vi "Add Node to Children.vi"(9 "Parent Path":string, 10 "Node Path":string, 11 "Tree Map In":T1) -> (1 "Path Invalid":bool, 3 "Tree Map Out":T1)   [LabVIEW 2019, in "Tree Map.lvlib"]
doc: "<b>Author:</b> Piotr Kruczkowski <PrimaryKey>\n<b>License:</b> NewBSD\n\nCopyright (c) 2019, National Instruments\nAll rights reserved.\n\nRedistribution and use in source and binary forms, with or without\nmodification, are permitted provided that the following conditions are met:\n1. Redistributions of source code must retain the above copyright\n notice, this list of conditions and the following disclaimer.\n2. Redistributions in binary form must reproduce the above copyright\n notice, this list of conditions and the following disclaimer in the\n documentation and/or other materials provided with the distribution.\n3. Neither the name of National Instruments nor the\n names of its contributors may be used to endorse or promote products\n derived from this software without specific prior written permission.\n\nTHIS SOFTWARE IS PROVIDED BY National Instruments ''AS IS'' AND ANY\nEXPRESS OR IMPLIED WARRANTIES, INCLUDING, BUT NOT LIMITED TO, THE IMPLIED\nWARRANTIES OF MERCHANTABILITY AND FITNESS FOR A PARTICULAR PURPOSE ARE\nDISCLAIMED. IN NO EVENT SHALL National Instruments BE LIABLE FOR ANY\nDIRECT, INDIRECT, INCIDENTAL, SPECIAL, EXEMPLARY, OR CONSEQUENTIAL DAMAGES\n(INCLUDING, BUT NOT LIMITED TO, PROCUREMENT OF SUBSTITUTE GOODS OR SERVICES;\nLOSS OF USE, DATA, OR PROFITS; OR BUSINESS INTERRUPTION) HOWEVER CAUSED AND\nON ANY THEORY OF LIABILITY, WHETHER IN CONTRACT, STRICT LIABILITY, OR TORT\n(INCLUDING NEGLIGENCE OR OTHERWISE) ARISING IN ANY WAY OUT OF THE USE OF THIS\nSOFTWARE, EVEN IF ADVISED OF THE POSSIBILITY OF SUCH DAMAGE."
uses:
  Tree Map.lvlib
  Tree Map Data.ctl
  <vilib>/Utility/miscctls.llb/LVMapReplaceAction.ctl
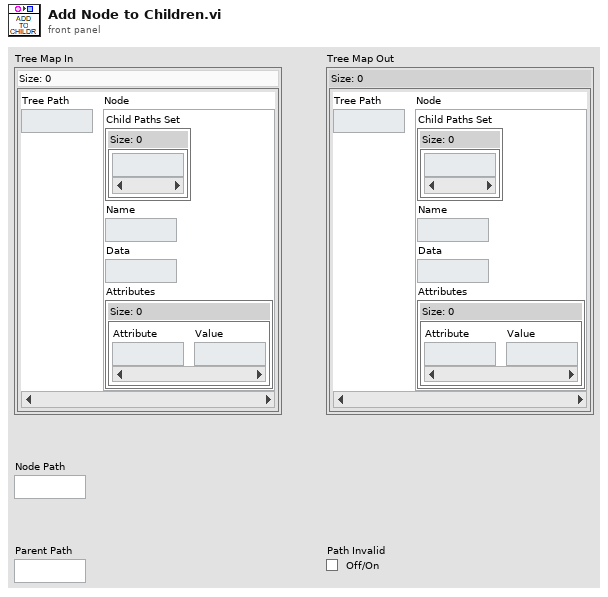
[diagram p1: front panel]
types:
  T1 = typedef "Tree Map.lvlib/Tree Map Data.ctl" = map{string, cluster{"Child Paths Set":set{string}, "Name":string, "Data":string, "Attributes":map{string, string}}}
  T2 = typedef "LVMapReplaceAction.ctl" = enum32{"Modify Entry only if found", "Add or Modify Entry", "Delete Entry"}
  T3 = cluster{"Child Paths Set":set{string}, "Name":string, "Data":string, "Attributes":map{string, string}}
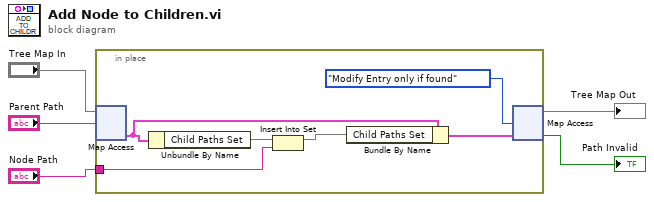
[diagram p0: block diagram]
diagram:
  n1 = in-place {
    in-place-border: "Node Path" -> [w11]
    # "Add the branch path as child of parent."
    n2 = in-place-map #1("Tree Map In", "Parent Path") -> (w8:T3)  [unwired: 1 in, 1 out]
    n3 = Unbundle By Name(w8) -> ("Child Paths Set"=w10:set{string})
    n4 = Insert Into Set(10:w11, 11:w10) -> (3:w9:set{string})  [unwired: 1 out]
    n5 = Bundle By Name(cluster=w8, "Child Paths Set"=w9) -> (w7:T3)
    n6 = in-place-map #1(w7, LVMapReplaceAction."Modify Entry only if found" ("action")) -> (→"Tree Map Out":T1, →"Path Invalid":bool)  [unwired: 1 out]
  }
